vi "Get Provided Interface and Service Class.vi"(8 "error in":errorcluster, 11 "instrument in":refnum<class "Session Factory.lvclass">) -> (0 "error out":errorcluster, 1 "service class":string, 2 "provided interface":string, 3 "instrument out":refnum<class "Session Factory.lvclass">)   [LabVIEW 2020, in "MeasurementLink niDigital.lvlib" / "Session Factory.lvclass"]
uses:
  Session Factory.lvclass
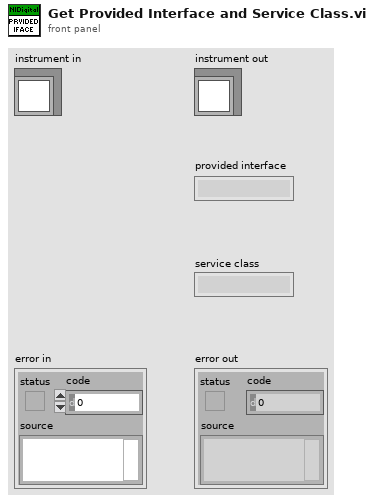
[diagram p1: front panel]
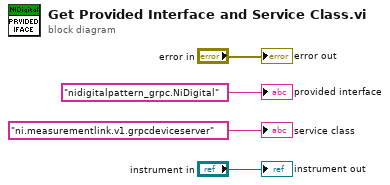
[diagram p0: block diagram]
diagram:
  "error out" <- "error in"
  "instrument out" <- "instrument in"
  "provided interface" <- "nidigitalpattern_grpc.NiDigital" ("provided interface")
  "service class" <- "ni.measurementlink.v1.grpcdeviceserver" ("service_class")
